vi "hw3_2.vi"() -> ()   [LabVIEW 2014]
panel:
  out "sorted":dbl[](graph)
  out "partially sorted":dbl[](graph)
  out "unsorted":dbl[](graph)
  out "sorted":dbl[](array[numeric])
  out "partially sorted":dbl[](array[numeric])
  out "unsorted":dbl[](array[numeric])
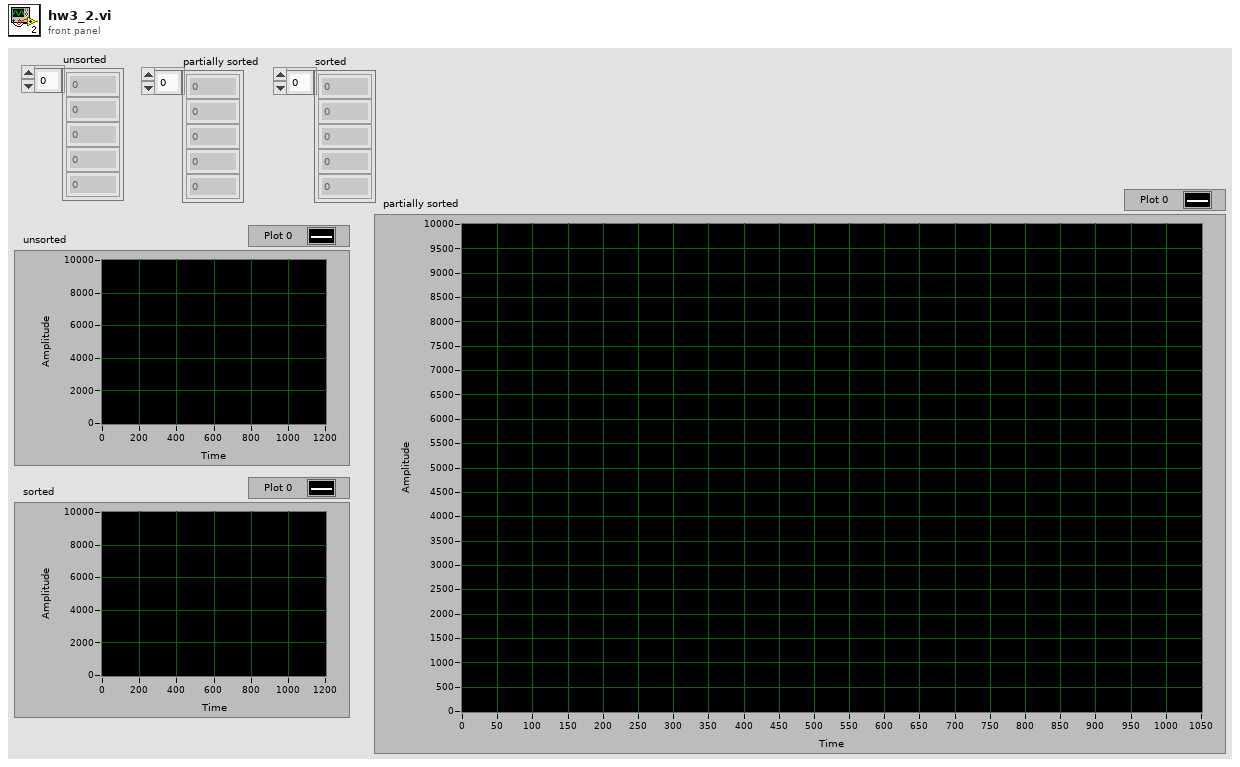
[diagram p1: front panel]
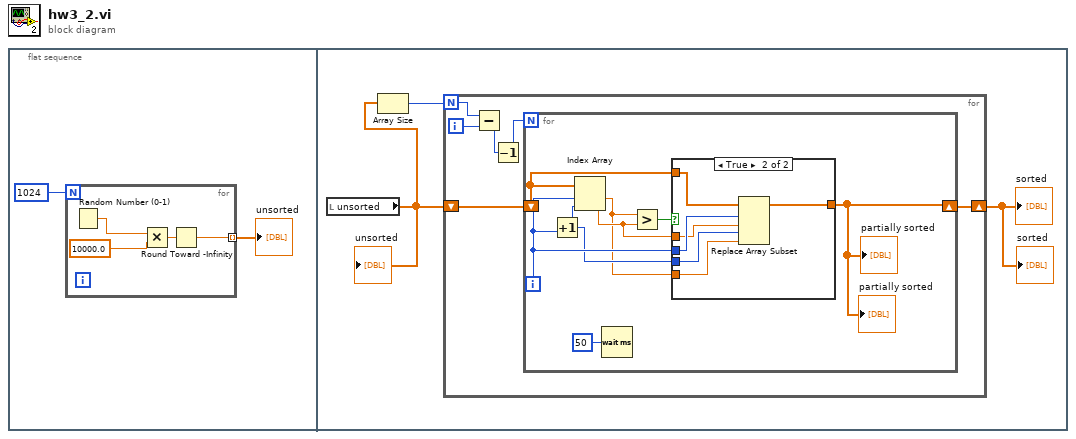
[diagram p0: block diagram]
diagram:
  n1 = flat-sequence {
    frame #0 {
      n2 = for {
        N: 1024 -> [_]
        tunnel: [w3] -> w1 mode=indexing
        n3 = Random Number (0-1)() -> (number: 0 to 1=w4:dbl)
        n4 = Multiply(x=w4, y=10000.0) -> (x*y=w6:dbl)
        n5 = Round Toward -Infinity(1:w6) -> (0:w3:dbl)
      }
      "unsorted" <- w1
    }
    frame #1 {
      n6 = local read "unsorted"() -> (w8:dbl[])
      "unsorted" <- w8
      n7 = Array Size(array=w8) -> (size(s)=w9:i32)
      n8 = for {
        N: w9 -> [w13]
        shift-right: [w14] -> w7
        shift-left: w8 -> [w15]
        i -> [w12]
        n9 = Subtract(x=w13, y=w12) -> (x-y=w11:i32)
        n10 = Decrement(x=w11) -> (x-1=w10:i32)
        n11 = for {
          N: w10 -> [_]
          shift-right: [w17] -> w14
          shift-left: w15 -> [w22]
          i -> [w21]
          n12 = Increment(x=w21) -> (x+1=w20:i32)
          n13 = Index Array(array=w22, index #1=w21, index #2=w20) -> (element #1=w18:dbl, element #2=w19:dbl)
          n14 = Wait (ms)(milliseconds to wait=u32 50) -> ()  [unwired: 1 out]
          n15 = Greater?(x=w18, y=w19) -> (0:w23:bool)
          n16 = case shown="True" w23 {
            tunnel: w22 -> [w24 w25]
            tunnel: w21 -> [_ w30]
            tunnel: w19 -> [_ w29]
            tunnel: w20 -> [_ w28]
            tunnel: w18 -> [_ w27]
            tunnel: [w24 w26] -> w17
            frame False {
            }
            frame True {
              n17 = Replace Array Subset(array=w25, new element #1=w29, index #1=w30, new element #2=w27, index #2=w28) -> (w26:dbl[])
            }
          }
          "partially sorted" <- w17
          "partially sorted" <- w17
        }
      }
      "sorted" <- w7
      "sorted" <- w7
    }
  }
